vi "Initialize From JSON.vi"(8 "error in (no error)":errorcluster, 9 "version":T1, 10 "json":string, 11 "DSF UDP Thread Configuration in":refnum<class "DSF UDP Thread Settings.lvclass">) -> (0 "error out":errorcluster, 3 "DSF UDP Thread Configuration out":refnum<class "DSF UDP Thread Settings.lvclass">)   [LabVIEW 2017, in "DSF Core.lvlib" / "DSF UDP Thread Settings.lvclass"]
uses:
  DSF UDP Thread Settings.lvclass
  Typedefs/DSF Version Info.ctl
  DSF UDP Thread Settings.lvclass/DSF UDP Thread Settings.ctl
  DSF Core.lvlib
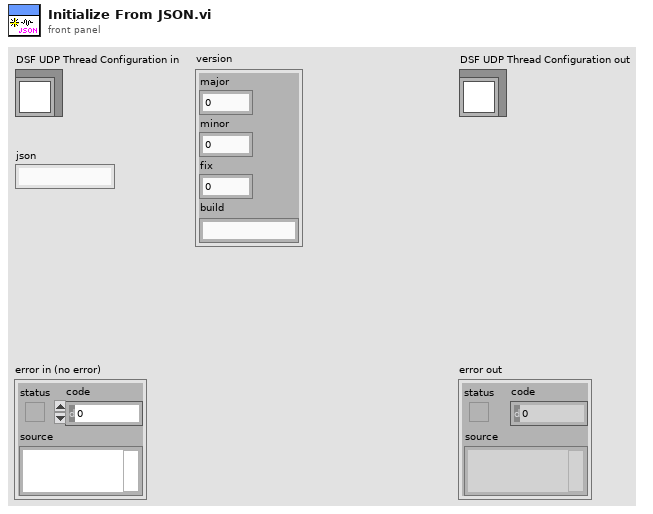
[diagram p1: front panel]
types:
  T1 = typedef "DSF Core.lvlib/DSF Version Info.ctl" = cluster{"major":u32, "minor":u32, "fix":u32, "build":string}
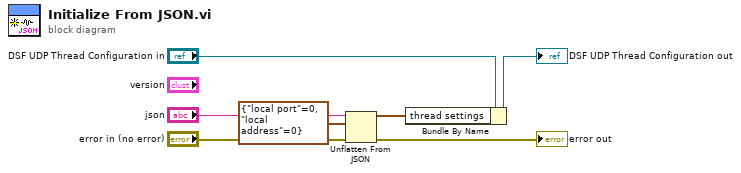
[diagram p0: block diagram]
diagram:
  n1 = Unflatten From JSON(JSON string="json", type and defaults=cluster{"local port":u16, "local address":u32} {"local port"=0, "local address"=0} ("thread settings"), error in (no error)="error in (no error)") -> (value=w1:cluster{"local port":u16, "local address":u32}, error out=→"error out":errorcluster)  [unwired: 4 in]
  n2 = Bundle By Name(cluster="DSF UDP Thread Configuration in", "thread settings"=w1) -> (→"DSF UDP Thread Configuration out":refnum<class "DSF UDP Thread Settings.lvclass">)
